vi "0x55_Progress_preparing_table_data.vi"(8 "error in":errorcluster, 10 "Param":cluster{"Номер табличного параметра":i32}, 11 "paramUnicorn 2":T2={"conParam"={"ReadIntParam"=TRUE, "ReadDescrParam"=FALSE, "ReadFloatParam"=TRUE, "debug"=FALSE, "ReadJSON"=TRUE, "IP_address"="192.168.1.216", "N_attempts"=3, "type_con"=enum."TCP", "MB_address"=1, "VISA"="COM1", "connection ID"=refnum, "nameDevices"="", "timeout"=3000, "port"=2000, "type_version"="0F0C0001", "baud_rate"=115200, "VersionControl"=TRUE, "TCP_conn"=TRUE, "WindowSize"=700}, "Param"={"NumParam"={"NTelem"=201, "NInt"=16, "NFloat"=10, "NTable"=2}, "ParamInt"=[{"ID"="Режим работы", "Num"=0, "Name"="", "Type"="", "Enum"="", "Desc"="", "Unit"="", "Access"="", "FormatStr"="", "Min"=0, "Max"=0}, {"ID"="", "Num"=0, "Name"="", "Type"="", "Enum"="", "Desc"="", "Unit"="", "Access"="", "FormatStr"="", "Min"=0, "Max"=0}, {"ID"="", "Num"=0, "Name"="", "Type"="", "Enum"="", "Desc"="", "Unit"="", "Access"="", "FormatStr"="", "Min"=0, "Max"=0}, {"ID"="", "Num"=0, "Name"="", "Type"="", "Enum"="", "Desc"="", "Unit"="", "Access"="", "FormatStr"="", "Min"=0, "Max"=0}, {"ID"="", "Num"=0, "Name"="", "Type"="", "Enum"="", "Desc"="", "Unit"="", "Access"="", "FormatStr"="", "Min"=0, "Max"=0}, {"ID"="", "Num"=0, "Name"="", "Type"="", "Enum"="", "Desc"="", "Unit"="", "Access"="", "FormatStr"="", "Min"=0, "Max"=0}, {"ID"="ModeWork", "Num"=0, "Name"="", "Type"="", "Enum"="", "Desc"="", "Unit"="", "Access"="", "FormatStr"="", "Min"=0, "Max"=0}], "Telemetry"=[], "Table"=[], "ParamFloat"=[]}}) -> (0 "error out":errorcluster, 1 "Cluster":T1, 2 "Ответ":string, 3 "paramUnicorn":T2={"conParam"={"ReadIntParam"=TRUE, "ReadDescrParam"=FALSE, "ReadFloatParam"=TRUE, "debug"=FALSE, "ReadJSON"=TRUE, "IP_address"="192.168.1.216", "N_attempts"=3, "type_con"=enum."TCP", "MB_address"=1, "VISA"="COM1", "connection ID"=refnum, "nameDevices"="", "timeout"=3000, "port"=2000, "type_version"="0F0C0001", "baud_rate"=115200, "VersionControl"=TRUE, "TCP_conn"=TRUE, "WindowSize"=700}, "Param"={"NumParam"={"NTelem"=201, "NInt"=16, "NFloat"=10, "NTable"=2}, "ParamInt"=[{"ID"="Режим работы", "Num"=0, "Name"="", "Type"="", "Enum"="", "Desc"="", "Unit"="", "Access"="", "FormatStr"="", "Min"=0, "Max"=0}, {"ID"="", "Num"=0, "Name"="", "Type"="", "Enum"="", "Desc"="", "Unit"="", "Access"="", "FormatStr"="", "Min"=0, "Max"=0}, {"ID"="", "Num"=0, "Name"="", "Type"="", "Enum"="", "Desc"="", "Unit"="", "Access"="", "FormatStr"="", "Min"=0, "Max"=0}, {"ID"="", "Num"=0, "Name"="", "Type"="", "Enum"="", "Desc"="", "Unit"="", "Access"="", "FormatStr"="", "Min"=0, "Max"=0}, {"ID"="", "Num"=0, "Name"="", "Type"="", "Enum"="", "Desc"="", "Unit"="", "Access"="", "FormatStr"="", "Min"=0, "Max"=0}, {"ID"="", "Num"=0, "Name"="", "Type"="", "Enum"="", "Desc"="", "Unit"="", "Access"="", "FormatStr"="", "Min"=0, "Max"=0}, {"ID"="ModeWork", "Num"=0, "Name"="", "Type"="", "Enum"="", "Desc"="", "Unit"="", "Access"="", "FormatStr"="", "Min"=0, "Max"=0}], "Telemetry"=[], "Table"=[], "ParamFloat"=[]}}, 5 "Сообщение об ошибке":bool)   [LabVIEW 2017, in "LV_Unicorn.lvlib"]
uses:
  LV_Unicorn.lvlib
  Control/unicorn_Param.ctl
  Control/unicorn_conn.ctl
  Control/unicorn_JSON.ctl
  Control/unicorn_ParamInt.ctl
  Control/unicorn_Telemetry.ctl
  Control/unicorn_Table.ctl
  Control/unicorn_ParamFloat.ctl
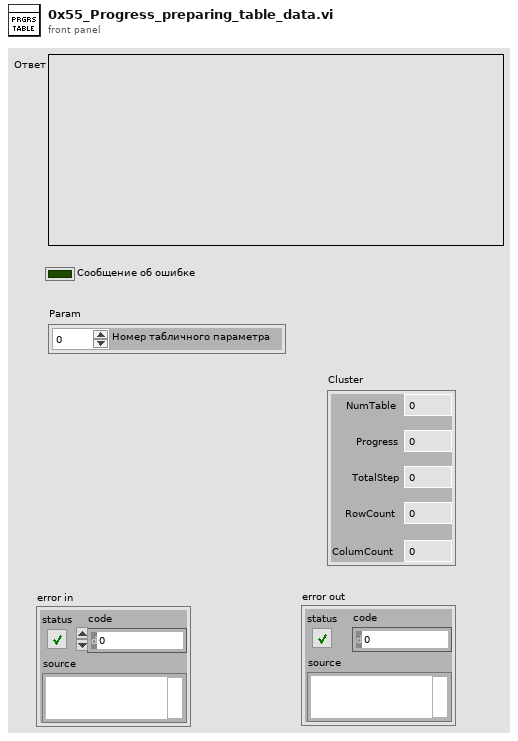
[diagram p1: front panel]
types:
  T1 = cluster{"NumTable":i32, "Progress":i32, "TotalStep":i32, "RowCount":i32, "ColumCount":i32}
  T2 = typedef "LV_Unicorn.lvlib/unicorn_Param.ctl" = cluster{"conParam":T3, "Param":T4}
  T3 = typedef "LV_Unicorn.lvlib/unicorn_conn.ctl" = cluster{"ReadIntParam":bool, "ReadDescrParam":bool, "ReadFloatParam":bool, "debug":bool, "ReadJSON":bool, "IP_address":string, "N_attempts":i32, "type_con":enum16{"Serial", "TCP"}, "MB_address":i32, "VISA":refnum<visa-resource-name>, "connection ID":refnum<k5>, "nameDevices":string, "timeout":i32, "port":u16, "type_version":string, "baud_rate":u32, "VersionControl":bool, "TCP_conn":bool, "WindowSize":i32}
  T4 = typedef "LV_Unicorn.lvlib/unicorn_JSON.ctl" = cluster{"NumParam":cluster{"NTelem":i32, "NInt":i32, "NFloat":i32, "NTable":i32}, "ParamInt":T5, "Telemetry":T6, "Table":T7, "ParamFloat":T8}
  T5 = typedef "LV_Unicorn.lvlib/unicorn_ParamInt.ctl" = cluster{"ID":string, "Num":i32, "Name":string, "Type":string, "Enum":string, "Desc":string, "Unit":string, "Access":string, "FormatStr":string, "Min":i32, "Max":i32}[]
  T6 = typedef "LV_Unicorn.lvlib/unicorn_Telemetry.ctl" = cluster{"ID":string, "Num":i32, "Name":string, "Desc":string, "Unit":string, "FormatStr":string, "Min":i32, "Max":i32}[]
  T7 = typedef "LV_Unicorn.lvlib/unicorn_Table.ctl" = cluster{"Num":i32, "Access":string, "ColumnCount":i32, "NeedParamPrepare":bool, "Columns":cluster{"Column":i32, "Desc":string, "Name":string}[], "DataType":string, "FormatStr":string, "ID":string, "Name":string, "RowCount":i32, "Rows":cluster{"Desc":string, "ID":string, "Max":i32, "Min":i32, "Name":string, "Row":i32, "Unit":string}[], "Type":string}[]
  T8 = typedef "LV_Unicorn.lvlib/unicorn_ParamFloat.ctl" = cluster{"ID":string, "Num":i32, "Name":string, "Type":string, "Enum":string, "Desc":string, "Unit":string, "Access":string, "FormatStr":string, "Min":sgl, "Max":sgl}[]
  T9 = cluster{"NumTable":i32, "Progress":i32, "Общее количество шагов для получения результата":i32, "Количество строк в подготовленном табличном параметре":i32, "Количество столбцов в подготовленном табличном параметре":i32}
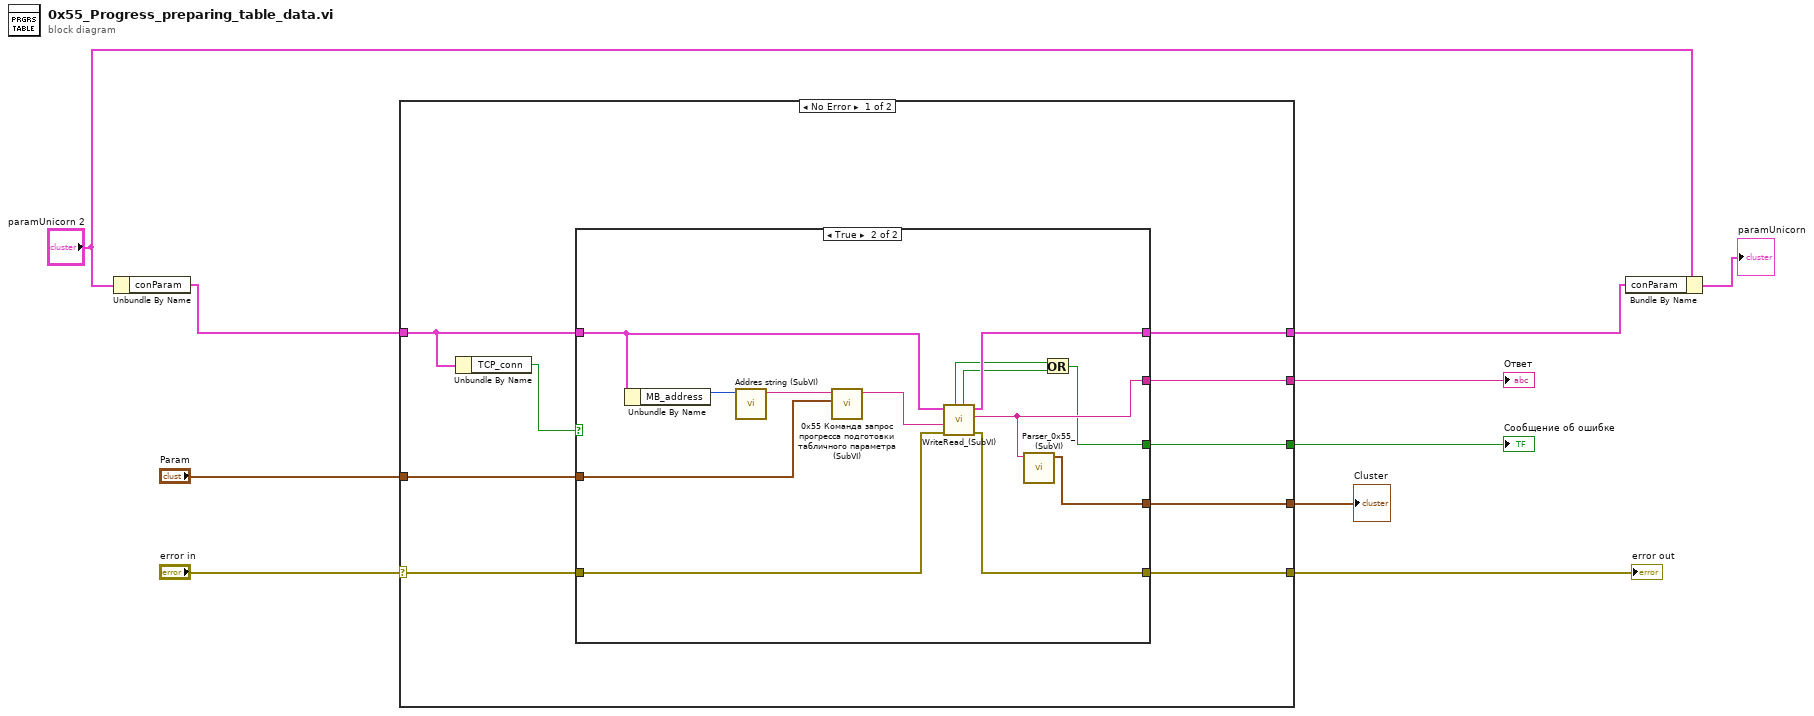
[diagram p0: block diagram]
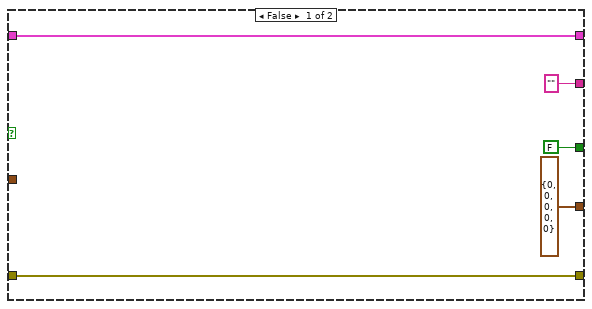
[diagram p2: hidden frame]
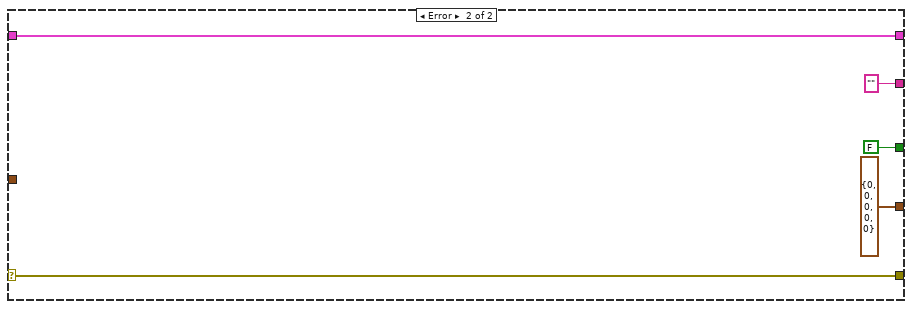
[diagram p3: hidden frame]
diagram:
  n1 = Unbundle By Name("paramUnicorn 2") -> ("conParam"=w7:T3)
  n2 = case shown="No Error" "error in" {
    selector: "error in" -> [w17 w41]
    tunnel: w7 -> [w13 w42]
    tunnel: [w19 w42] -> w5
    tunnel: [w18 w41] -> w10
    tunnel: "Param" -> [w16 _]
    tunnel: [w15 "" ("Ответ")] -> w3
    tunnel: [w14 FALSE ("Сообщение об ошибке")] -> w2
    tunnel: [w11 T9 {"NumTable"=0, "Progress"=0, "Общее количество шагов для получения результата"=0, "Количество строк в подготовленном табличном параметре"=0, "Количество столбцов в подготовленном табличном параметре"=0} ("Cluster")] -> w1
    frame No Error {
      n3 = Unbundle By Name(w13) -> ("TCP_conn"=w12:bool)
      n4 = case shown="True" w12 {
        tunnel: [w24 w37] -> w19
        tunnel: [w21 w36] -> w18
        tunnel: w17 -> [w21 w35]
        tunnel: w13 -> [w24 w34]
        tunnel: w16 -> [_ w31]
        tunnel: ["" ("Ответ") w29] -> w15
        tunnel: [FALSE ("Сообщение об ошибке") w25] -> w14
        tunnel: [T9 {"NumTable"=0, "Progress"=0, "Общее количество шагов для получения результата"=0, "Количество строк в подготовленном табличном параметре"=0, "Количество столбцов в подготовленном табличном параметре"=0} ("Cluster") w28] -> w11
        frame False {
        }
        frame True {
          n5 = Unbundle By Name(w34) -> ("MB_address"=w33:i32)
          n6 = call "Addres string (SubVI).vi"("Адрес"=w33) -> ("String"=w30:string)  [unwired: 10 in]
          n7 = call "0x55 Команда запрос прогресса подготовки табличного параметра (SubVI).vi"("Parameters"=w31, "String in"=w30) -> ("String out"=w32:string)  [unwired: 9 in]
          n8 = call "WriteRead_(SubVI).vi"("error in"=w35, "Запрос"=w32, "ParamIn"=w34) -> ("error out"=w36:errorcluster, "Ответ"=w29:string, "ParamOut"=w37:T3, "ErrorMessage"=w26:bool, "GatewayTimeout"=w27:bool)  [unwired: 4 in]
          n9 = call "Parser_0x55_(SubVI).vi"("String in"=w29) -> ("Cluster"=w28:T9)  [unwired: 9 in, 1 out]
          n10 = Or(x=w27, y=w26) -> (x .or. y?=w25:bool)
        }
      }
    }
    frame Error {
    }
  }
  "error out" <- w10
  "Сообщение об ошибке" <- w2
  "Ответ" <- w3
  "Cluster" <- w1
  n11 = Bundle By Name(cluster="paramUnicorn 2", "conParam"=w5) -> (→"paramUnicorn":T2)
